vi "3-12.vi"() -> ()   [LabVIEW 2022 SP3]
panel:
  out "数组":dbl[](array[numeric])
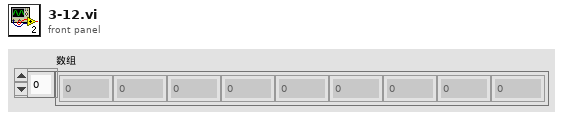
[diagram p1: front panel]
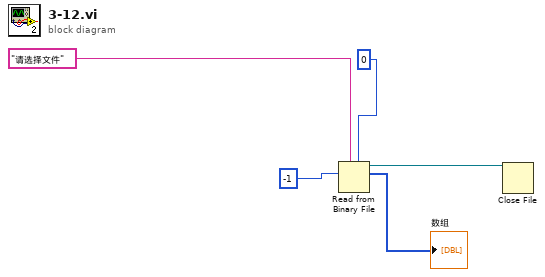
[diagram p0: block diagram]
diagram:
  n1 = Read from Binary File(5:0 ("总数(1)"), 7:"请选择文件", 10:-1) -> (2:→"数组":i32[], 3:w1:refnum<file>)  [unwired: 3 in, 2 out]
  n2 = Close File(refnum=w1) -> ()  [unwired: 1 in, 2 out]
